vi "eWriteName and eReadName.vi"(0 "Handle In":i32, 1 "Read Name":string="AIN0", 5 "Write Name":string="DAC0", 9 "Write Value":dbl=1.5 format="%.6f", 11 "error in":errorcluster) -> (4 "Handle Out":i32, 10 "Read Value":dbl format="%.6f", 15 "error out":errorcluster)   [LabVIEW 2024]
panel:
  out "Error String":string
  # "The VIs in the \\Functions folder are the basic function calls from the LJM library and\nare set up as sub-VIs that need to be called by some parent VI.  Those LJM functions\ncan do everything including combined writes and reads in a single packet.\n\nThis utility VI does 2 LJM calls ... a call to eReadName followed by a call to\neWriteName ... which will result in 2 low-level modbus transactions.  This can be\ndone more efficiently with eNames which will use 1 modbus transaction if\npossible, but this utility VI might be a simpler option when max speed is not important."
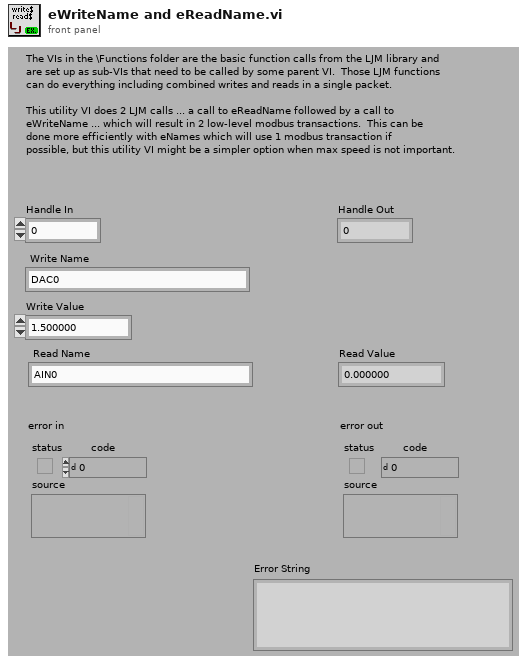
[diagram p1: front panel]
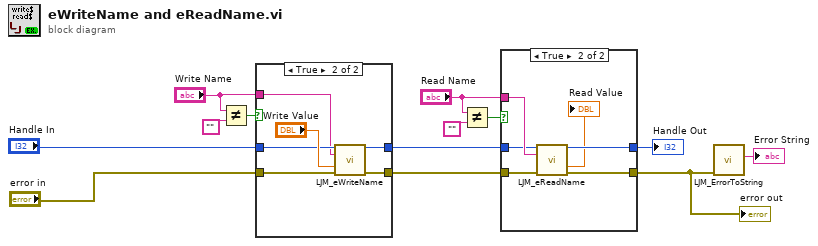
[diagram p0: block diagram]
diagram:
  n1 = Not Equal?(x="Write Name", y="") -> (x != y?=w4:bool)
  n2 = case shown="True" w4 {
    tunnel: "Handle In" -> [w15 w20]
    tunnel: "error in" -> [w14 w19]
    tunnel: [w14 w18] -> w10
    tunnel: [w15 w17] -> w9
    tunnel: "Write Name" -> [_ w16]
    frame False {
    }
    frame True {
      n3 = call "LJM_eWriteName.vi"("Handle In"=w20, "Name"=w16, "Value"="Write Value", "error in"=w19) -> ("Handle Out"=w17:i32, "error out"=w18:errorcluster)  [unwired: 10 in]
    }
  }
  n4 = Not Equal?(x="Read Name", y="") -> (x != y?=w2:bool)
  n5 = case shown="True" w2 {
    tunnel: "Read Name" -> [_ w29]
    tunnel: w10 -> [w22 w28]
    tunnel: w9 -> [w23 w27]
    tunnel: [w23 w26] -> w8
    tunnel: [w22 w25] -> w7
    frame False {
    }
    frame True {
      n6 = call "LJM_eReadName.vi"("Handle In"=w27, "Name"=w29, "error in"=w28) -> ("Handle Out"=w26:i32, "Value"=→"Read Value":dbl, "error out"=w25:errorcluster)  [unwired: 10 in]
    }
  }
  "error out" <- w7
  "Handle Out" <- w8
  n7 = call "LJM_ErrorToString.vi"("error in"=w7) -> ("String"=→"Error String":string)  [unwired: 10 in]
